vi "Write Execute Test VIs.vi"(8 "error in (no error)":errorcluster, 10 "Execute Test VIs":path[](array[path]), 11 "TestBench in":refnum<class "TestBench.lvclass">) -> (0 "error out":errorcluster, 3 "TestBench out":refnum<class "TestBench.lvclass">)   [LabVIEW 2019, in "TestBench.lvlib" / "TestBench.lvclass"]
uses:
  TestBench.lvclass
  TestBench.lvclass/TestBench.ctl
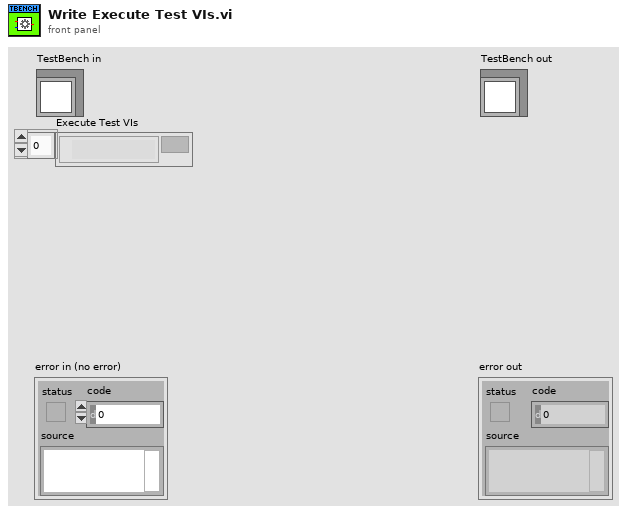
[diagram p1: front panel]
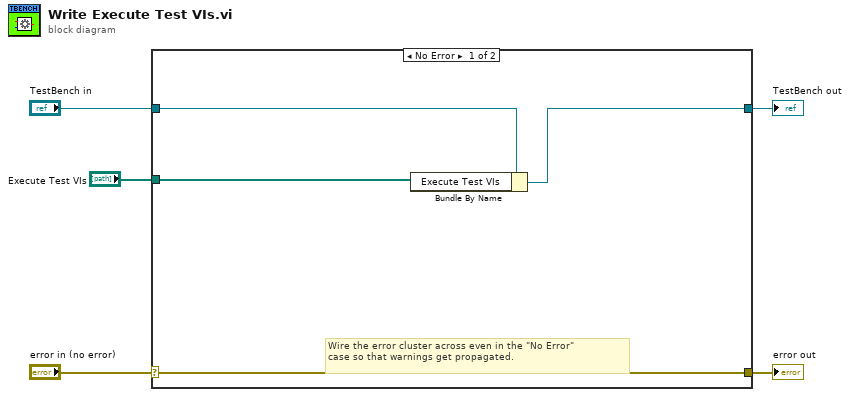
[diagram p0: block diagram]
diagram:
  n1 = case shown="No Error" "error in (no error)" {
    selector: "error in (no error)" -> [w9 w11]
    tunnel: [w9 w11] -> w4
    tunnel: [w7 w10] -> w2
    tunnel: "TestBench in" -> [w8 w10]
    tunnel: "Execute Test VIs" -> [w6 _]
    frame No Error {
      # "Wire the error cluster across even in the \"No Error\"\ncase so that warnings get propagated."
      n2 = Bundle By Name(cluster=w8, "Execute Test VIs"=w6) -> (w7:refnum<class "TestBench.lvclass">)
    }
    frame Error {
    }
  }
  "error out" <- w4
  "TestBench out" <- w2
